vi "Write State.vi"(8 "error in (no error)":errorcluster, 10 "State":u16, 11 "State Machine in":refnum<class "State Machine.lvclass">) -> (0 "error out":errorcluster, 3 "State Machine out":refnum<class "State Machine.lvclass">)   [LabVIEW 2018, in "State Machine.lvclass"]
uses:
  State Machine.lvclass
  State Machine.lvclass/State Machine.ctl
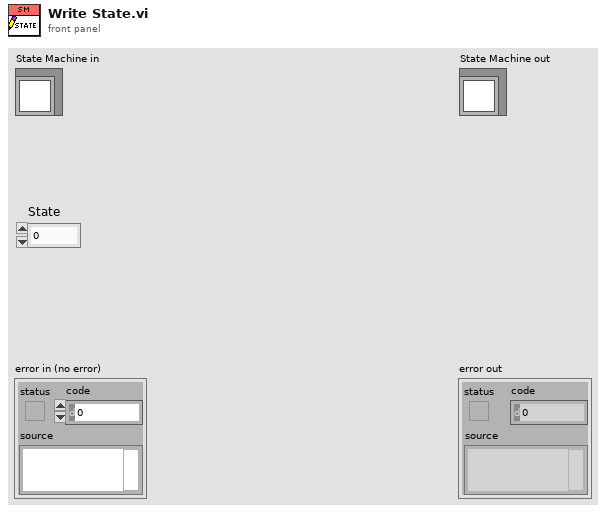
[diagram p1: front panel]
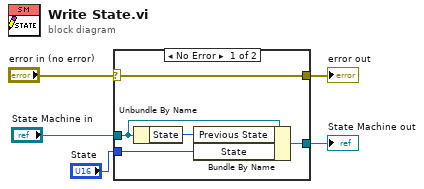
[diagram p0: block diagram]
diagram:
  n1 = case shown="No Error" "error in (no error)" {
    selector: "error in (no error)" -> [w10 w11]
    tunnel: [w10 w11] -> w4
    tunnel: [w9 w12] -> w2
    tunnel: "State Machine in" -> [w8 w12]
    tunnel: "State" -> [w6 _]
    frame No Error {
      n2 = Unbundle By Name(w8) -> ("State"=w7:u16)
      n3 = Bundle By Name(cluster=w8, "Previous State"=w7, "State"=w6) -> (w9:refnum<class "State Machine.lvclass">)
    }
    frame Error {
    }
  }
  "error out" <- w4
  "State Machine out" <- w2
